vi "detectVarablesFromIP.vi"(3 "error in (no error)":errorcluster, 4 "PortIP":string, 5 "VISA resource name":refnum<visa-resource-name>="COM1" caption="端口号") -> (0 "error out":errorcluster, 1 "Data":T1[](array[typedef]), 2 "VISA resource name 2":refnum<visa-resource-name>="COM1" caption="端口号")   [LabVIEW 2010]
uses:
  types/OutputDataFormat.ctl
  types/VarableID.ctl
  main/AmmeterGlobalCostants.vi
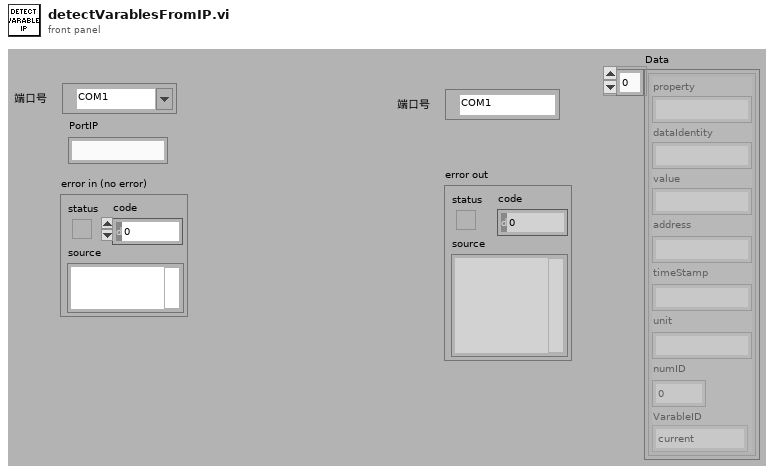
[diagram p1: front panel]
types:
  T1 = typedef "OutputDataFormat.ctl" = cluster{"property":string, "dataIdentity":string, "value":string, "address":string, "timeStamp":string, "unit":string, "numID":i32, "VarableID":T2}
  T2 = typedef "VarableID.ctl" = enum16{"current", "power", "PF", "voltage"}
  T3 = typedef "VarableStruct.ctl" = cluster{"Name":string, "StorageRefnum":refnum<file>, "Command":string, "IsDetecting":bool, "VarableID":T2}
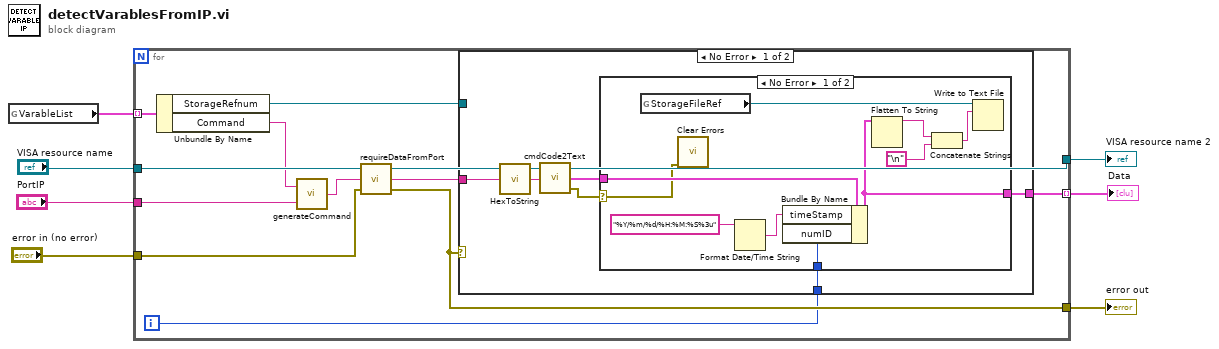
[diagram p0: block diagram]
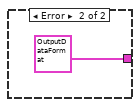
[diagram p2: hidden frame]
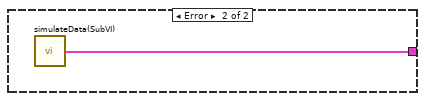
[diagram p3: hidden frame]
diagram:
  n1 = global read "AmmeterGlobalCostants.vi" "VarableList"() -> (w7:T3[])
  n2 = for "For循环" {
    tunnel: w7 -> [w16] mode=indexing
    tunnel: "VISA resource name" -> [w19]
    tunnel: [w18] -> w5
    tunnel: "error in (no error)" -> [w14]
    tunnel: [w13] -> w3
    tunnel: "PortIP" -> [w12]
    tunnel: [w10] -> w1 mode=indexing
    i -> [w9]
    n3 = Unbundle By Name(w16) -> ("StorageRefnum"=w17:refnum<file>, "Command"=w8:string)
    n4 = call "generateCommand.vi"("IP"=w12, "CommandProtoType"=w8) -> ("Command"=w11:string)
    n5 = call "requireDataFromPort.vi"("error in (no error)"=w14, "Command"=w11, "VISA resource name"=w19) -> ("error out"=w13:errorcluster, "Data"=w15:string, "VISA resource name 2"=w18:refnum<visa-resource-name>)
    n6 = case shown="No Error" w13 {
      tunnel: w17 -> [_ _]
      tunnel: w15 -> [w25 _]
      tunnel: [w23 w37] -> w10
      tunnel: w9 -> [w21 _]
      frame No Error {
        n7 = call "HexToString.vi"("input Hex"=w25) -> ("output string"=w24:string)
        n8 = call "cmdCode2Text.vi"("CommandCode"=w24) -> ("error out"=w20:errorcluster, "CommandText"=w22:T1)  [unwired: 3 in]
        n9 = case shown="No Error" w20 {
          selector: w20 -> [w26 _]
          tunnel: [w32 T1 {"property"="", "dataIdentity"="", "value"="", "address"="", "timeStamp"="", "unit"="", "numID"=0, "VarableID"=enum."current"} ("CommandText")] -> w23
          tunnel: w22 -> [w31 _]
          tunnel: w21 -> [w28 _]
          frame No Error {
            n10 = global read "AmmeterGlobalCostants.vi" "StorageFileRef"() -> (w27:refnum<file>)
            n11 = call <vilib>:"Clear Errors.vi"("error in (no error)"=w26) -> ()  [unwired: 6 in, 1 out]
            n12 = Format Date/Time String(time format string (%c)="%Y/%m/%d/%H:%M:%S%3u") -> (date/time string=w29:string)  [unwired: 2 in]
            n13 = Bundle By Name(cluster=w31, "timeStamp"=w29, "numID"=w28) -> (w32:T1)
            n14 = Flatten To String(anything=w32) -> (data string=w33:string)  [unwired: 3 in, 2 out]
            n15 = Concatenate Strings(w33, "\n") -> (w34:string)
            n16 = Write to Text File(file (use dialog)=w27, text=w34) -> ()  [unwired: 2 in, 3 out]
          }
          frame Error {
          }
        }
      }
      frame Error {
        n17 = call "simulateData(SubVI).vi"() -> ("output cluster"=w37:T1)
      }
    }
  }
  "VISA resource name 2" <- w5
  "error out" <- w3
  "Data" <- w1
